vi "Advantech Data Processing.vi"(8 "Error In":errorcluster, 10 "TC Coefficients":T1, 11 "Raw Data":dbl[](array[numeric])) -> (0 "Error Out":errorcluster, 1 "Advantech Data Output":dbl[](array[numeric]), 2 "Advantech Data List Headers":string[][](array[string]), 3 "Advantech":T2)   [LabVIEW 2018]
uses:
  Type Definitions/Advantech DAQ.ctl
  Trunk/Utility/Type Definitions/UTILITY TC Coefficients.ctl
  Trunk/Utility/Type Definitions/UTILITY TC Coefficients Selector.ctl
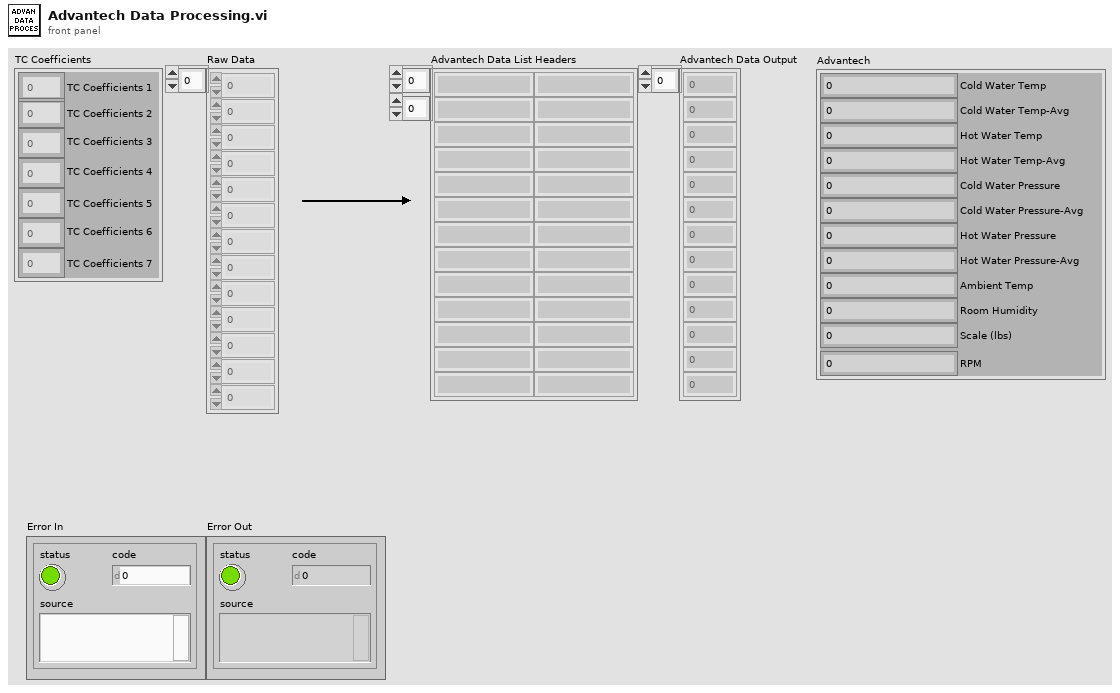
[diagram p1: front panel]
types:
  T1 = typedef "UTILITY TC Coefficients.ctl" = cluster{"TC Coefficients 1":dbl[], "TC Coefficients 2":dbl[], "TC Coefficients 3":dbl[], "TC Coefficients 4":dbl[], "TC Coefficients 5":dbl[], "TC Coefficients 6":dbl[], "TC Coefficients 7":dbl[]}
  T2 = typedef "Advantech DAQ.ctl" = cluster{"Cold Water Pressure":dbl, "Hot Water Pressure":dbl, "Cold Water Temp":dbl, "Hot Water Temp":dbl, "Ambient Temp":dbl, "Room Humidity":dbl, "Scale (lbs)":dbl, "RPM":dbl, "Cold Water Temp-Avg":dbl, "Hot Water Temp-Avg":dbl, "Cold Water Pressure-Avg":dbl, "Hot Water Pressure-Avg":dbl}
  T3 = typedef "UTILITY TC Coefficients Selector.ctl" = enum16{"TC1", "TC2", "TC3", "TC4", "TC5", "TC6", "TC7"}
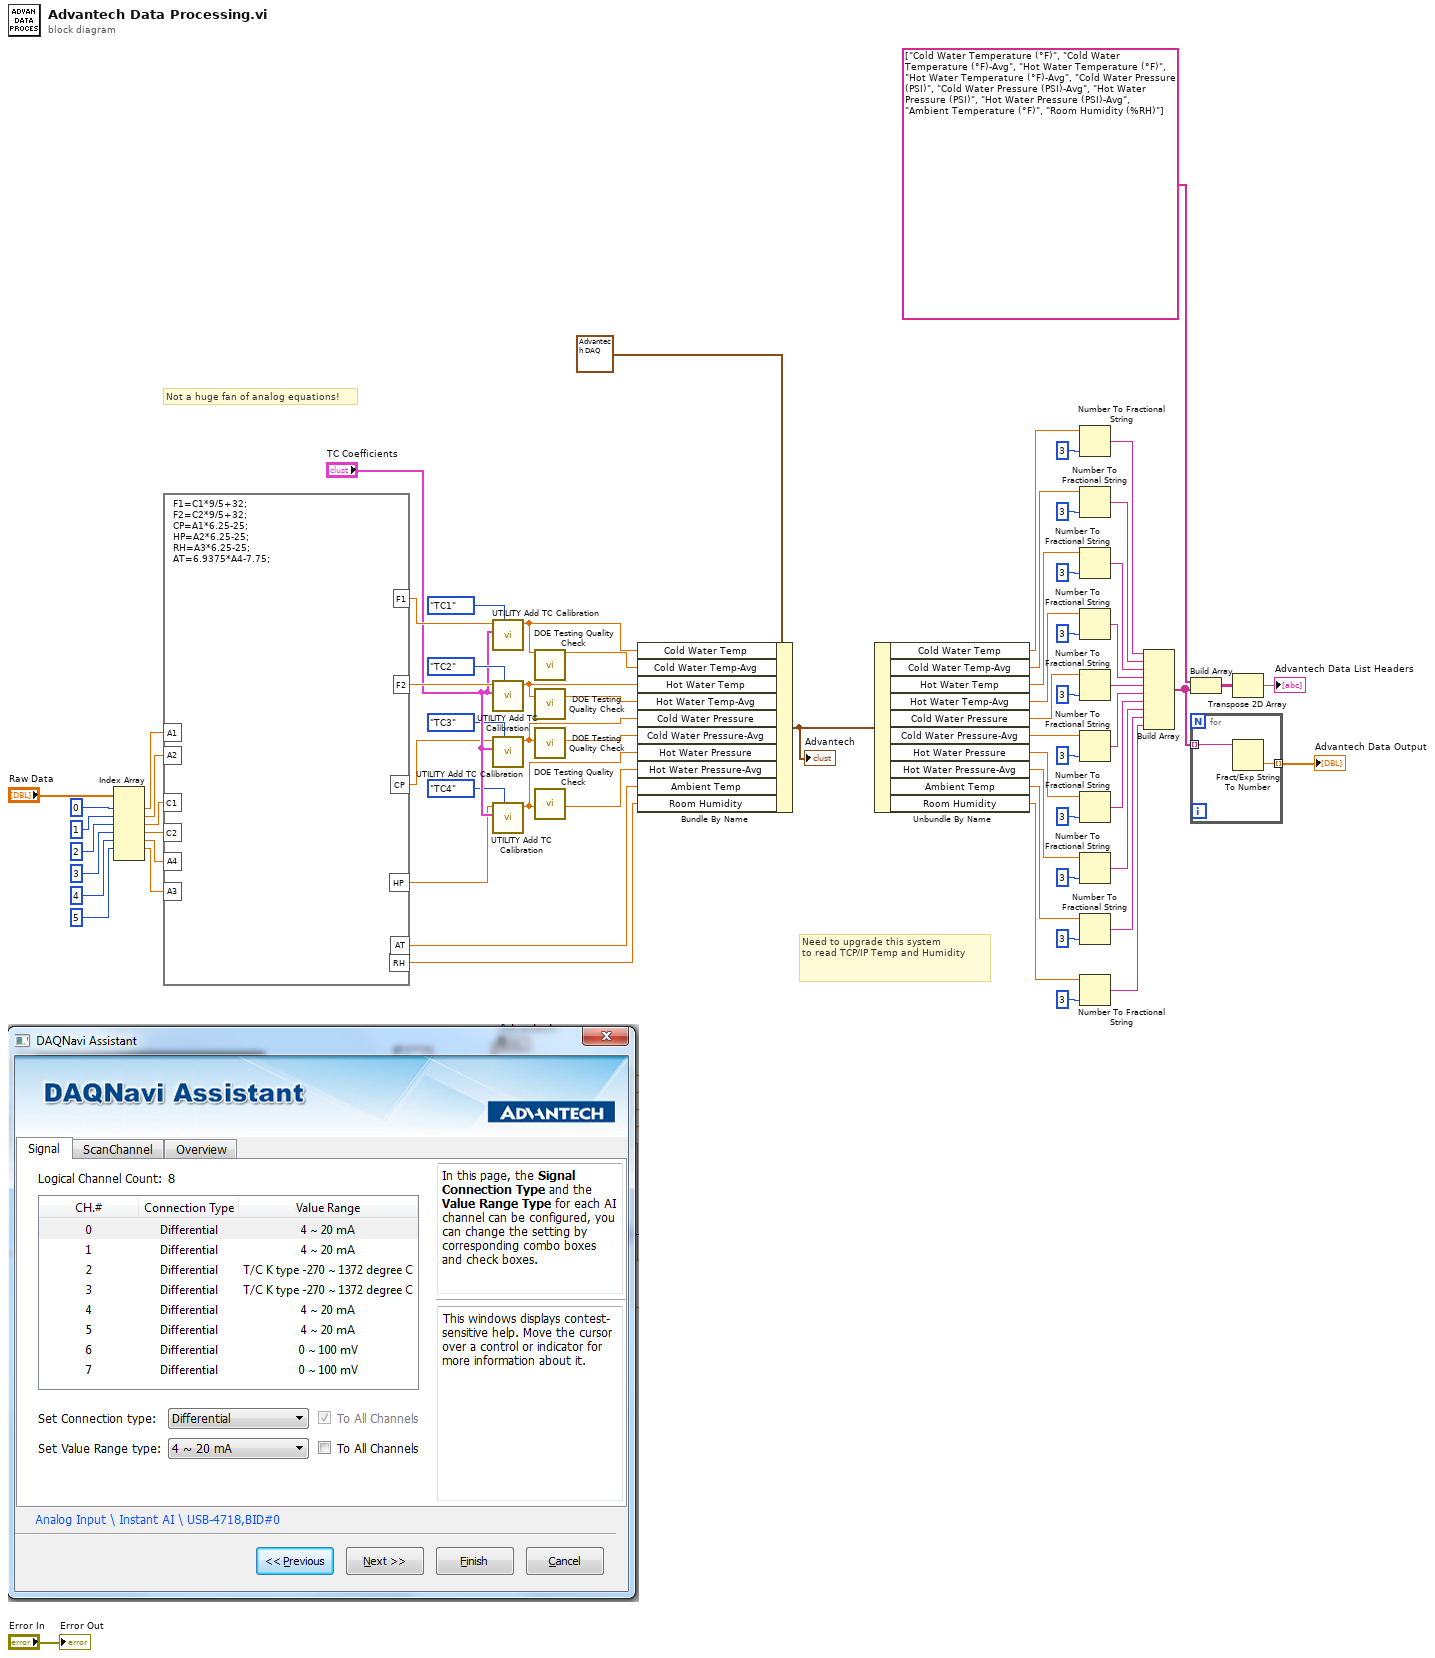
[diagram p0: block diagram]
diagram:
  # "Need to upgrade this system\nto read TCP/IP Temp and Humidity"
  # "Not a huge fan of analog equations!"
  n1 = Index Array(array="Raw Data", index #1=0 ("index"), index #2=1 ("index"), index #3=2 ("index"), index #4=3 ("index"), index #5=4 ("index"), index #6=5 ("index")) -> (element #1=w46:dbl, element #2=w45:dbl, element #3=w44:dbl, element #4=w43:dbl, element #5=w42:dbl, element #6=w41:dbl)  [unwired: 1 in, 1 out]
  n2 = formula code="F1=C1*9/5+32;\nF2=C2*9/5+32;\nCP=A1*6.25-25;\nHP=A2*6.25-25;\nRH=A3*6.25-25;\nAT=6.9375*A4-7.75;"("C1"=w44, "C2"=w43, "A1"=w46, "A2"=w45, "A3"=w41, "A4"=w42) -> ("F1"=w67:dbl, "F2"=w68:dbl, "CP"=w29:dbl, "HP"=w28:dbl, "RH"=w38:dbl, "AT"=w39:dbl)
  n3 = call "UTILITY Add TC Calibration.vi"("Enum"=UTILITY_TC_Coefficients_Selector."TC1", "TC Coefficients"="TC Coefficients", "Non Cal Temp"=w67) -> ("Calibrated Temp"=w12:dbl)  [unwired: 8 in]
  n4 = call "UTILITY Add TC Calibration.vi"("Enum"=UTILITY_TC_Coefficients_Selector."TC2", "TC Coefficients"="TC Coefficients", "Non Cal Temp"=w68) -> ("Calibrated Temp"=w10:dbl)  [unwired: 8 in]
  n5 = call "UTILITY Add TC Calibration.vi"("Enum"=UTILITY_TC_Coefficients_Selector."TC3", "TC Coefficients"="TC Coefficients", "Non Cal Temp"=w29) -> ("Calibrated Temp"=w8:dbl)  [unwired: 8 in]
  n6 = call "UTILITY Add TC Calibration.vi"("Enum"=UTILITY_TC_Coefficients_Selector."TC4", "TC Coefficients"="TC Coefficients", "Non Cal Temp"=w28) -> ("Calibrated Temp"=w6:dbl)  [unwired: 8 in]
  n7 = call "DOE Testing Quality Check.vi"("Cold Water Temp Input"=w12) -> ("Cold Water Temp Avg"=w11:dbl)  [unwired: 14 in, 4 out]
  n8 = call "DOE Testing Quality Check.vi"("Hot Water Temp Input"=w10) -> ("Hot Water Temp Avg"=w9:dbl)  [unwired: 14 in, 4 out]
  n9 = call "DOE Testing Quality Check.vi"("Cold Water Pressure Input"=w8) -> ("Cold Water Pressure Avg"=w7:dbl)  [unwired: 14 in, 4 out]
  n10 = call "DOE Testing Quality Check.vi"("Hot Water Pressure Input"=w6) -> ("Hot Water Pressure Avg"=w5:dbl)  [unwired: 14 in, 4 out]
  n11 = Bundle By Name(cluster=T2 {"Cold Water Pressure"=0.0, "Hot Water Pressure"=0.0, "Cold Water Temp"=0.0, "Hot Water Temp"=0.0, "Ambient Temp"=0.0, "Room Humidity"=0.0, "Scale (lbs)"=0.0, "RPM"=0.0, "Cold Water Temp-Avg"=0.0, "Hot Water Temp-Avg"=0.0, "Cold Water Pressure-Avg"=0.0, "Hot Water Pressure-Avg"=0.0} ("Advantech 2"), "Cold Water Temp"=w12, "Cold Water Temp-Avg"=w11, "Hot Water Temp"=w10, "Hot Water Temp-Avg"=w9, "Cold Water Pressure"=w8, "Cold Water Pressure-Avg"=w7, "Hot Water Pressure"=w6, "Hot Water Pressure-Avg"=w5, "Ambient Temp"=w39, "Room Humidity"=w38) -> (w37:T2)
  "Advantech" <- w37
  n12 = Unbundle By Name(w37) -> ("Cold Water Temp"=w24:dbl, "Cold Water Temp-Avg"=w4:dbl, "Hot Water Temp"=w23:dbl, "Hot Water Temp-Avg"=w3:dbl, "Cold Water Pressure"=w22:dbl, "Cold Water Pressure-Avg"=w2:dbl, "Hot Water Pressure"=w21:dbl, "Hot Water Pressure-Avg"=w1:dbl, "Ambient Temp"=w55:dbl, "Room Humidity"=w56:dbl)
  n13 = Number To Fractional String(number=w24, precision (6)=i16 3) -> (F-format string=w57:string)  [unwired: 2 in]
  n14 = Number To Fractional String(number=w4, precision (6)=i16 3) -> (F-format string=w16:string)  [unwired: 2 in]
  n15 = Number To Fractional String(number=w23, precision (6)=i16 3) -> (F-format string=w58:string)  [unwired: 2 in]
  n16 = Number To Fractional String(number=w3, precision (6)=i16 3) -> (F-format string=w15:string)  [unwired: 2 in]
  n17 = Number To Fractional String(number=w22, precision (6)=i16 3) -> (F-format string=w59:string)  [unwired: 2 in]
  n18 = Number To Fractional String(number=w2, precision (6)=i16 3) -> (F-format string=w14:string)  [unwired: 2 in]
  n19 = Number To Fractional String(number=w21, precision (6)=i16 3) -> (F-format string=w60:string)  [unwired: 2 in]
  n20 = Number To Fractional String(number=w1, precision (6)=i16 3) -> (F-format string=w13:string)  [unwired: 2 in]
  n21 = Number To Fractional String(number=w55, precision (6)=i16 3) -> (F-format string=w61:string)  [unwired: 2 in]
  n22 = Number To Fractional String(number=w56, precision (6)=i16 3) -> (F-format string=w62:string)  [unwired: 2 in]
  n23 = Build Array(w57, w16, w58, w15, w59, w14, w60, w13, w61, w62) -> (w65:string[])
  n24 = Build Array(string[] ["Cold Water Temperature (°F)", "Cold Water Temperature (°F)-Avg", "Hot Water Temperature (°F)", "Hot Water Temperature (°F)-Avg", "Cold Water Pressure (PSI)", "Cold Water Pressure (PSI)-Avg", "Hot Water Pressure (PSI)", "Hot Water Pressure (PSI)-Avg", "Ambient Temperature (°F)", "Room Humidity (%RH)"], w65) -> (w63:string[][])
  n25 = for {
    tunnel: w65 -> [w72] mode=indexing
    tunnel: [w71] -> w66 mode=indexing
    n26 = Fract/Exp String To Number(string=w72) -> (number=w71:dbl)  [unwired: 3 in, 1 out]
  }
  "Advantech Data Output" <- w66
  n27 = Transpose 2D Array(2D array=w63) -> (transposed array=→"Advantech Data List Headers":string[][])
  "Error Out" <- "Error In"
